vi "Overlay GD & T.vi"(8 "error in (no error)":errorcluster, 10 "Overlay details in":T1, 11 "Image in":T2) -> (0 "error out":errorcluster, 1 "Overlay coordinates":cluster{"X":dbl, "Y":dbl}[](array[cluster]), 2 "Text origin":cluster{"X":dbl, "Y":dbl}, 3 "Image out":T2)   [LabVIEW 2019]
uses:
  <vilib>/vision/Image Controls.llb/IMAQ Image.ctl
  Controls/GD&T overlay.ctl
  <vilib>/vision/NI_Vision_Development_Module.lvlib
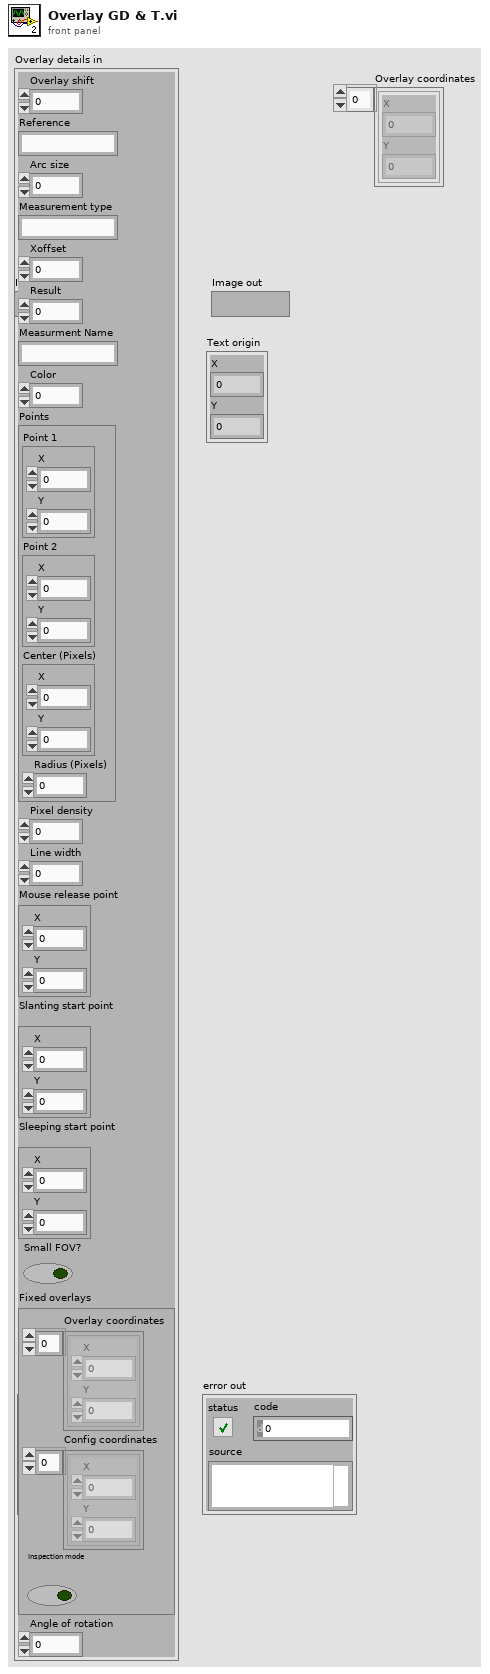
[diagram p1: front panel]
types:
  T1 = typedef "GD&T overlay.ctl" = cluster{"Overlay shift":dbl, "Reference":string, "Arc size":dbl, "Measurement type":string, "Xoffset":i32, "Result":sgl, "Measurment Name":string, "Color":u32, "Points":cluster{"Point 1":cluster{"X":sgl, "Y":sgl}, "Point 2":cluster{"X":sgl, "Y":sgl}, "Center (Pixels)":cluster{"X":sgl, "Y":sgl}, "Radius (Pixels)":dbl}, "Pixel density":dbl, "Line width":i32, "Mouse release point":cluster{"X":dbl, "Y":dbl}, "Slanting start point":cluster{"X":dbl, "Y":dbl}, "Sleeping start point":cluster{"X":dbl, "Y":dbl}, "Small FOV?":bool, "Fixed overlays":cluster{"Overlay coordinates":cluster{"X":dbl, "Y":dbl}[], "Config coordinates":cluster{"X":dbl, "Y":dbl}[], "Inspection mode":bool}, "Angle of rotation":dbl}
  T2 = typedef "IMAQ Image.ctl" = refnum<image>
  T3 = cluster{"Point 1":cluster{"X":sgl, "Y":sgl}, "Point 2":cluster{"X":sgl, "Y":sgl}}
  T4 = cluster{"Point 1":cluster{"X":sgl, "Y":sgl}, "Point 2":cluster{"X":sgl, "Y":sgl}, "Center (Pixels)":cluster{"X":sgl, "Y":sgl}, "Radius (Pixels)":dbl}
  T5 = cluster{"Feature":cluster{"X":dbl, "Y":dbl}[], "Directing points":cluster{"X":dbl, "Y":dbl}[], "Bounding box (symbols)":cluster{"X":dbl, "Y":dbl}[], "Symbols":cluster{"X":dbl, "Y":dbl}[], "Bounding box (Results)":cluster{"X":dbl, "Y":dbl}[], "Results":cluster{"X":dbl, "Y":dbl}[], "Bounding box (Reference)":cluster{"X":dbl, "Y":dbl}[], "Reference":cluster{"X":dbl, "Y":dbl}[]}
  T6 = cluster{"Center (Pixels)":cluster{"X":sgl, "Y":sgl}, "Radius (Pixels)":dbl}
  T7 = cluster{"Overlay coordinates":cluster{"X":dbl, "Y":dbl}[], "Config coordinates":cluster{"X":dbl, "Y":dbl}[], "Inspection mode":bool}
  T8 = cluster{"Overlay coordinates":cluster{"X":dbl, "Y":dbl}[], "Config coordinates":cluster{"X":dbl, "Y":dbl}[], "Inspection mode?":bool}
  T9 = enum16{"User-specified Font", "Application Font", "System Font", "Dialog Font"}
  T10 = cluster{"Desired Font (Application)":enum16{"User-specified Font", "Application Font", "System Font", "Dialog Font"}, "[User-specified Font]":cluster{"Font Name":string, "Size":i16, "Strikeout?":bool, "Italic?":bool, "Underline?":bool, "Outline?":bool, "Shadow?":bool, "Bold?":bool, "Rotation Angle":dbl}, "Horizontal Alignment":i16, "Vertical Alignment":i16}
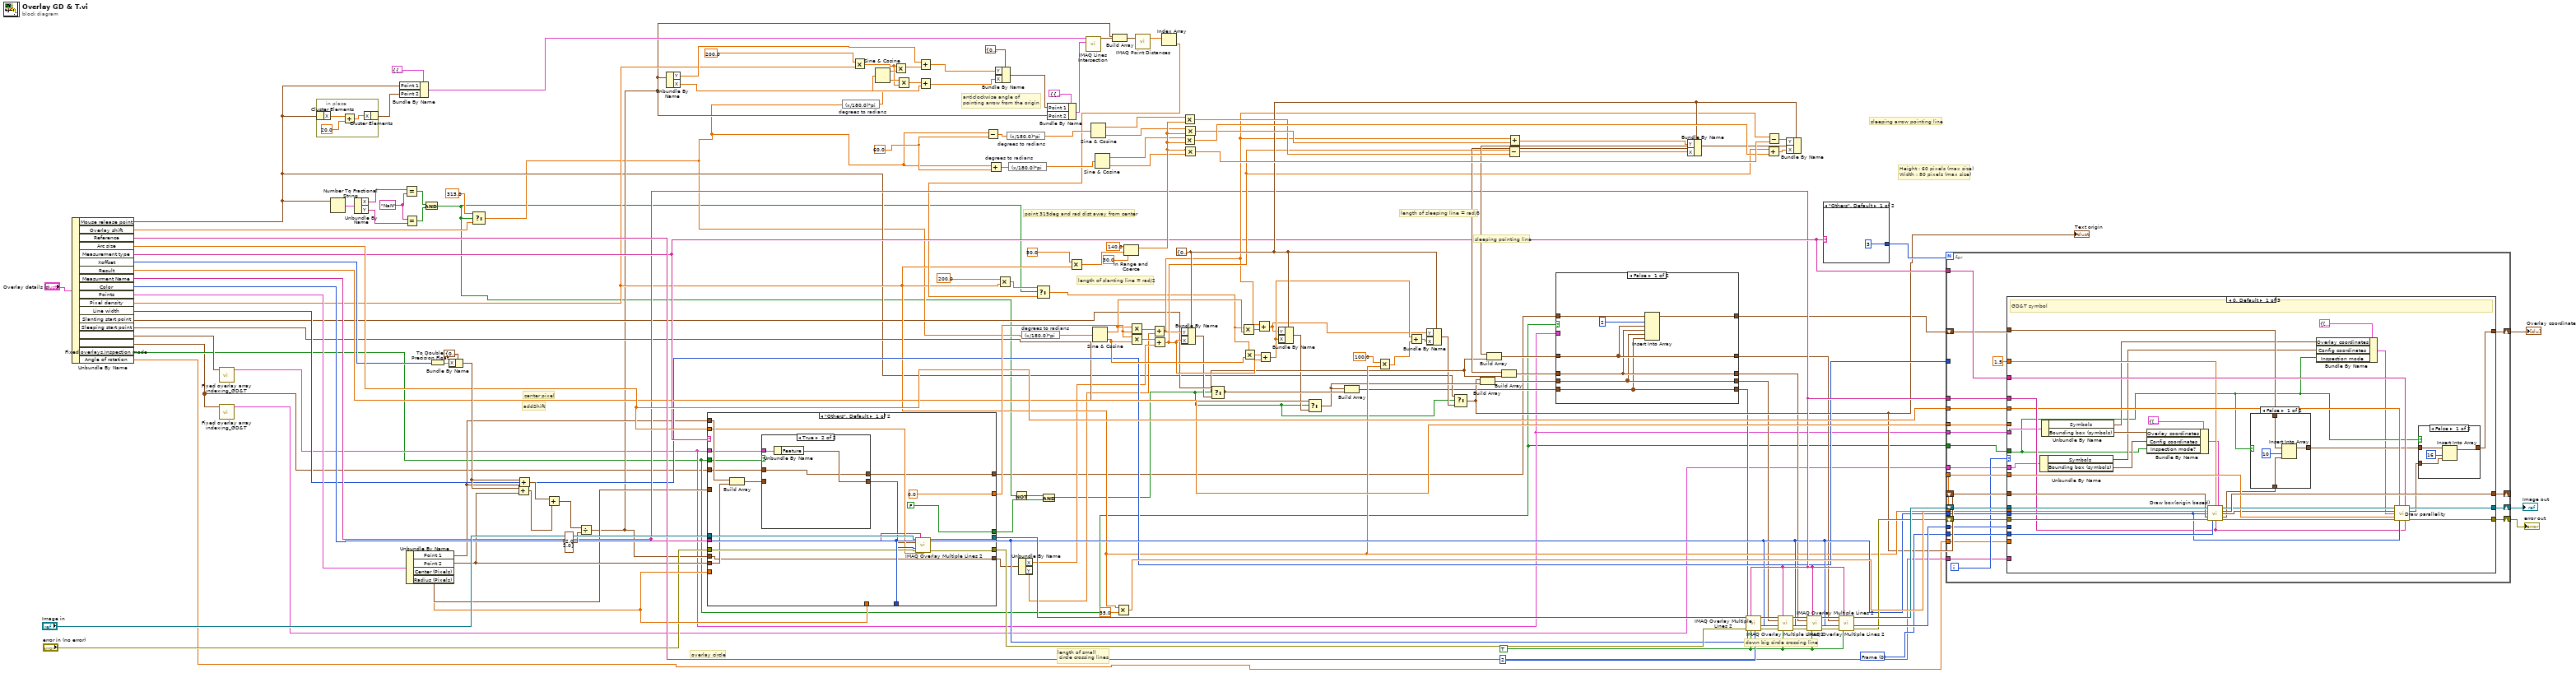
[diagram p0: block diagram]
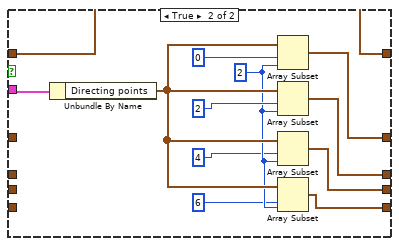
[diagram p2: hidden frame]
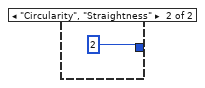
[diagram p3: hidden frame]
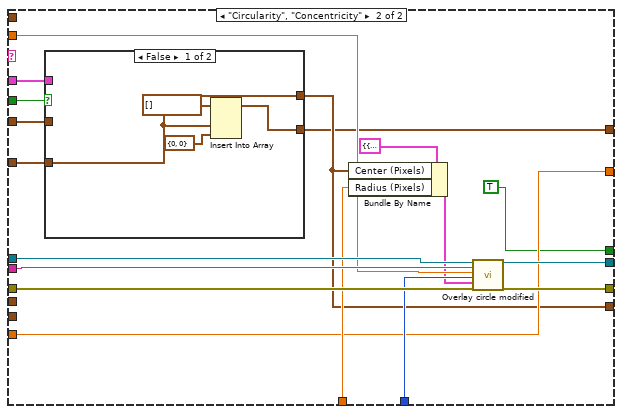
[diagram p5: hidden frame]
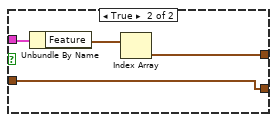
[diagram p6: hidden frame]
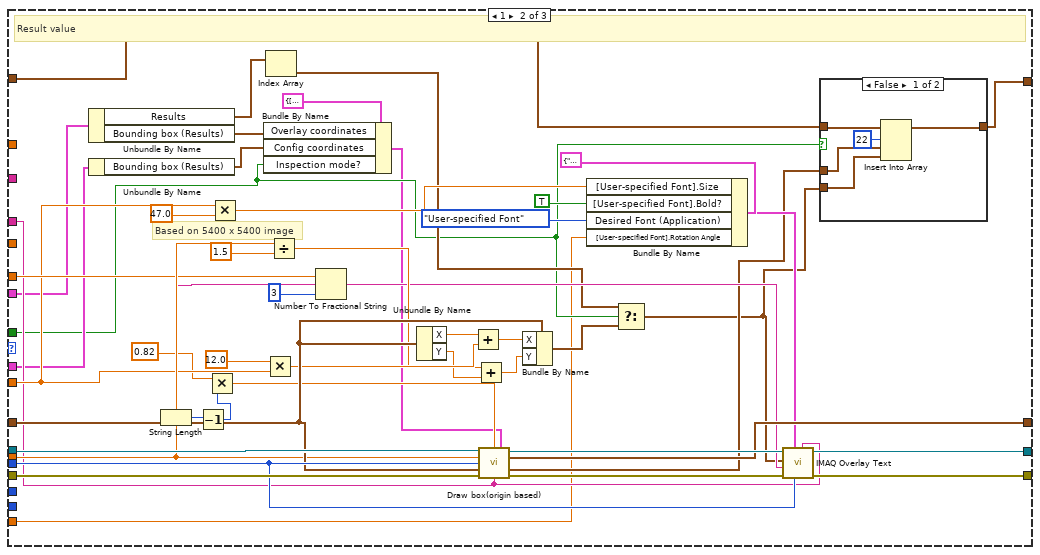
[diagram p9: hidden frame]
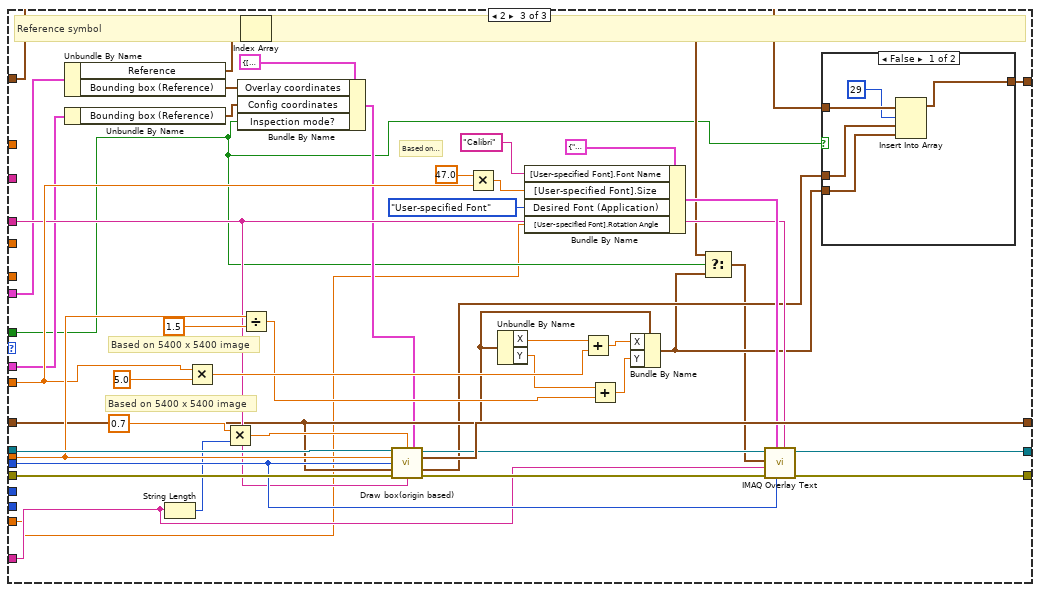
[diagram p11: hidden frame]
diagram:
  w71 = "NaN" ("y")
  w150 = u32 2 ("Width")
  w149 = TRUE ("Maintain Width?")
  w117 = 60.0
  w106 = u32 0 items=["Frame", "Fill"] ("Drawing Mode (Frame)")
  w132 = cluster{"X":sgl, "Y":sgl} {"X"=0.0, "Y"=0.0} ("Point 1")
  # "Height : 60 pixels (max size)\nWidth : 80 pixels (max size)"
  # "length of sleeping line = rad/8"
  # "point 315deg and rad dist away from center"
  # "length of slanting line = rad/2"
  # "length of small\n circle crossing lines"
  # "anticlockwise angle of\npointing arrow from the origin"
  # "sleeping arrow pointing line"
  # "sleeping pointing line"
  # "down big circle crossing line"
  # "addShift"
  # "center pixel"
  # "overlay circle"
  n1 = Unbundle By Name("Overlay details in") -> ("Mouse release point"=w26:cluster{"X":dbl, "Y":dbl}, "Overlay shift"=w21:dbl, "Reference"=w83:string, "Arc size"=w82:dbl, "Measurement type"=w81:string, "Xoffset"=w80:i32, "Result"=w79:sgl, "Measurment Name"=w78:string, "Color"=w77:u32, "Points"=w76:T4, "Pixel density"=w43:dbl, "Line width"=w75:i32, "Slanting start point"=w41:cluster{"X":dbl, "Y":dbl}, "Sleeping start point"=w38:cluster{"X":dbl, "Y":dbl}, "Fixed overlays.Overlay coordinates"=w17:cluster{"X":dbl, "Y":dbl}[], "Fixed overlays.Config coordinates"=w5:cluster{"X":dbl, "Y":dbl}[], "Fixed overlays.Inspection mode"=w6:bool, "Angle of rotation"=w1:dbl)
  n2 = call "Fixed overlay array indexing_GD&T.vi"("Overlay coordinates"=w17) -> ("Overlay coordinates cluster"=w7:T5)  [unwired: 10 in]
  n3 = call "Fixed overlay array indexing_GD&T.vi"("Overlay coordinates"=w5) -> ("Overlay coordinates cluster"=w4:T5)  [unwired: 10 in]
  n4 = in-place {
    n5 = in-place-cluster #1(w26) -> ("X"=w153:dbl)
    n6 = Add(x=w153, y=20.0) -> (x+y=w151:dbl)
    n7 = in-place-cluster #1("X"=w151) -> (w66:cluster{"X":dbl, "Y":dbl})
  }
  n8 = Number To Fractional String(number=w26) -> (F-format string=w74:cluster{"X":string, "Y":string})  [unwired: 3 in]
  n9 = Unbundle By Name(w74) -> ("X"=w73:string, "Y"=w72:string)
  n10 = Bundle By Name(cluster=T3 {"Point 1"={"X"=0.0, "Y"=0.0}, "Point 2"={"X"=0.0, "Y"=0.0}} ("Line 1"), "Point 1"=w26, "Point 2"=w66) -> (w65:T3)
  n11 = Equal?(x=w73, y=w71) -> (x = y?=w70:bool)
  n12 = Equal?(x=w71, y=w72) -> (x = y?=w69:bool)
  n13 = Unbundle By Name(w76) -> ("Point 1"=w68:cluster{"X":sgl, "Y":sgl}, "Point 2"=w35:cluster{"X":sgl, "Y":sgl}, "Center (Pixels)"=w34:cluster{"X":sgl, "Y":sgl}, "Radius (Pixels)"=w33:dbl)
  n14 = And(x=w70, y=w69) -> (x .and. y?=w19:bool)
  n15 = To Double Precision Float(number=w80) -> (double precision float=w97:dbl)
  n16 = Bundle By Name(cluster=cluster{"X":sgl, "Y":sgl} {"X"=0.0, "Y"=0.0} ("Angle.Point 2a"), "X"=w97) -> (w98:cluster{"X":sgl, "Y":sgl})
  n17 = Select(t=315.0, s=w19, f=w21) -> (s? t:f=w20:dbl)
  n18 = Add(x=w98, y=w35) -> (x+y=w102:cluster{"X":sgl, "Y":sgl})
  n19 = Add(x=w98, y=w68) -> (x+y=w101:cluster{"X":sgl, "Y":sgl})
  n20 = Add(x=w101, y=w102) -> (x+y=w99:cluster{"X":sgl, "Y":sgl})
  n21 = Divide(x=w99, y=cluster{"X":sgl, "Y":sgl} {"X"=2.0, "Y"=2.0}) -> (x/y=w28:cluster{"X":sgl, "Y":sgl})
  n22 = Unbundle By Name(w28) -> ("Y"=w61:sgl, "X"=w56:sgl)
  n23 = case shown="\"Others\", Default" w81 {
    tunnel: w33 -> [_ w183]
    tunnel: [sgl 0.0 w183] -> w116
    tunnel: "error in (no error)" -> [w171 w193]
    tunnel: [w170 w192] -> w146
    tunnel: "Image in" -> [w168 w191]
    tunnel: [w167 w190] -> w148
    tunnel: w78 -> [w163 w189]
    tunnel: w82 -> [w164 w188]
    tunnel: w77 -> [w169 w187]
    tunnel: w34 -> [_ w181]
    tunnel: w33 -> [_ w185]
    tunnel: w68 -> [w166 _]
    tunnel: w35 -> [w165 _]
    tunnel: [FALSE TRUE] -> w24
    tunnel: w28 -> [w160 _]
    tunnel: [w160 w180] -> w31
    tunnel: w6 -> [w157 w179]
    tunnel: w7 -> [w155 w178]
    tunnel: w5 -> [w154 w177]
    tunnel: [w156 w176] -> w8
    frame "Others", Default {
      n24 = Build Array(w166, w165) -> (w159:cluster{"X":sgl, "Y":sgl}[])
      n25 = case shown="True" w157 {
        tunnel: w159 -> [w172 _]
        tunnel: [w172 w174] -> w158
        tunnel: [w172 w173] -> w156
        tunnel: w155 -> [_ w175]
        tunnel: w154 -> [_ w173]
        frame False {
        }
        frame True {
          n26 = Unbundle By Name(w175) -> ("Feature"=w174:cluster{"X":dbl, "Y":dbl}[])
        }
      }
      n27 = call "IMAQ Overlay Multiple Lines 2"("Image"=w168, "Group"=w163, "Line End Points"=w158, "Color"=w169, "error in (no error)"=w171, "Width"=w164) -> ("Image Out"=w167:T2, "error out"=w170:errorcluster)  [unwired: 8 in]
    }
    frame "Circularity", "Concentricity" {
      n28 = case shown="False" w179 {
        tunnel: w181 -> [w197 _]
        tunnel: [w197 w199] -> w180
        tunnel: w178 -> [_ w201]
        tunnel: [w195 w198] -> w176
        tunnel: w177 -> [_ w198]
        frame False {
          n29 = Insert Into Array(array=cluster{"X":sgl, "Y":sgl}[] [], new element #1=w197, new element #2=cluster{"X":i32, "Y":i32} {"X"=0, "Y"=0} ("Center (Pixels)")) -> (w195:cluster{"X":sgl, "Y":sgl}[])  [unwired: 1 in]
        }
        frame True {
          n30 = Unbundle By Name(w201) -> ("Feature"=w200:cluster{"X":dbl, "Y":dbl}[])
          n31 = Index Array(array=w200) -> (element=w199:cluster{"X":dbl, "Y":dbl})  [unwired: 1 in]
        }
      }
      n32 = Bundle By Name(cluster=T6 {"Center (Pixels)"={"X"=0.0, "Y"=0.0}, "Radius (Pixels)"=0.0} ("Circle center"), "Center (Pixels)"=w180, "Radius (Pixels)"=w185) -> (w184:T6)
      n33 = call "Overlay circle modified.vi"("Image In"=w191, "Measurment Name"=w189, "Overlay width"=w188, "Overlay color"=w187, "Circle center"=w184, "error in (no error)"=w193) -> ("Image out"=w190:T2, "error out"=w192:errorcluster)  [unwired: 12 in]
    }
  }
  n34 = expression code="(x/180.0)*pi" "degrees to radians"(w20) -> (w47:dbl)
  n35 = Multiply(x=sgl 200.0, y=w43) -> (x*y=w58:dbl)
  n36 = Sine & Cosine(0:w47) -> (1:w62:dbl, 2:w59:dbl)
  n37 = Multiply(x=w58, y=w62) -> (x*y=w60:dbl)
  n38 = Multiply(x=w59, y=w58) -> (x*y=w57:dbl)
  n39 = Add(x=w61, y=w60) -> (x+y=w54:dbl)
  n40 = Add(x=w57, y=w56) -> (x+y=w53:dbl)
  n41 = Subtract(x=w20, y=w117) -> (x-y=w118:dbl)
  n42 = Add(x=w20, y=w117) -> (x+y=w119:dbl)
  n43 = Bundle By Name(cluster=cluster{"X":sgl, "Y":sgl} {"X"=0.0, "Y"=0.0} ("x/y"), "Y"=w54, "X"=w53) -> (w52:cluster{"X":sgl, "Y":sgl})
  n44 = Multiply(x=200.0 ("t"), y=w43) -> (x*y=w42:dbl)
  n45 = expression code="(x/180.0)*pi" "degrees to radians"(w118) -> (w124:dbl)
  n46 = expression code="(x/180.0)*pi" "degrees to radians"(w119) -> (w125:dbl)
  n47 = Not(x=w19) -> (.not. x?=w18:bool)
  n48 = Unbundle By Name(w31) -> ("X"=w30:dbl, "Y"=w29:dbl)
  n49 = expression code="(x/180.0)*pi" "degrees to radians"(w20) -> (w85:dbl)
  n50 = And(x=w18, y=w24) -> (x .and. y?=w23:bool)
  n51 = Bundle By Name(cluster=T3 {"Point 1"={"X"=0.0, "Y"=0.0}, "Point 2"={"X"=0.0, "Y"=0.0}} ("Line 1"), "Point 1"=w52, "Point 2"=w28) -> (w51:T3)
  n52 = Multiply(x=sgl 50.0, y=w43) -> (x*y=w141:dbl)
  n53 = call "IMAQ Lines Intersection"("Line 2"=w51, "Line 1"=w65) -> ("Intersection Point"=w50:cluster{"X":sgl, "Y":sgl})  [unwired: 7 in, 2 out]
  n54 = Sine & Cosine(0:w124) -> (1:w120:dbl, 2:w121:dbl)
  n55 = Sine & Cosine(0:w85) -> (1:w86:dbl, 2:w87:dbl)
  n56 = Sine & Cosine(0:w125) -> (1:w122:dbl, 2:w123:dbl)
  n57 = Build Array(w28, w50) -> (w49:cluster{"X":sgl, "Y":sgl}[])
  n58 = Multiply(x=w43, y=35.0) -> (x*y=w107:dbl)
  n59 = In Range and Coerce(upper limit=140.0, x=w141, lower limit=30.0) -> (coerced(x)=w144:dbl)  [unwired: 1 out]
  n60 = Multiply(x=w86, y=w116) -> (x*y=w94:dbl)
  n61 = Multiply(x=w116, y=w87) -> (x*y=w95:dbl)
  n62 = call "IMAQ Point Distances"("Points"=w49) -> ("Distances"=w48:sgl[])  [unwired: 4 in, 1 out]
  n63 = Add(x=w94, y=w29) -> (x+y=w130:dbl)
  n64 = Add(x=w95, y=w30) -> (x+y=w131:dbl)
  n65 = Index Array(array=w48) -> (element=w45:sgl)  [unwired: 1 in]
  n66 = Select(t=w42, s=w19, f=w45) -> (s? t:f=w46:dbl)
  n67 = Bundle By Name(cluster=w132, "Y"=w130, "X"=w131) -> (w40:cluster{"X":sgl, "Y":sgl})
  n68 = Multiply(x=w120, y=w144) -> (x*y=w135:dbl)
  n69 = Multiply(x=w122, y=w144) -> (x*y=w137:dbl)
  n70 = Multiply(x=w121, y=w144) -> (x*y=w136:dbl)
  n71 = Multiply(x=w144, y=w123) -> (x*y=w138:dbl)
  n72 = Select(t=w41, s=w23, f=w40) -> (s? t:f=w39:cluster{"X":dbl, "Y":dbl})
  n73 = Multiply(x=w46, y=w86) -> (x*y=w88:dbl)
  n74 = Multiply(x=w46, y=w87) -> (x*y=w89:dbl)
  n75 = Add(x=w130, y=w88) -> (x+y=w92:dbl)
  n76 = Add(x=w89, y=w131) -> (x+y=w93:dbl)
  n77 = Bundle By Name(cluster=w132, "Y"=w92, "X"=w93) -> (w37:cluster{"X":sgl, "Y":sgl})
  n78 = Select(t=w38, s=w23, f=w37) -> (s? t:f=w36:cluster{"X":dbl, "Y":dbl})
  n79 = Build Array(w36, w39) -> (w10:cluster{"X":dbl, "Y":dbl}[])
  n80 = Multiply(x=100.0, y=w43) -> (x*y=w90:dbl)
  n81 = Add(x=w93, y=w90) -> (x+y=w91:dbl)
  n82 = Bundle By Name(cluster=w132, "Y"=w92, "X"=w91) -> (w27:cluster{"X":sgl, "Y":sgl})
  n83 = Select(t=w26, s=w23, f=w27) -> (s? t:f=w25:cluster{"X":dbl, "Y":dbl})
  "Text origin" <- w25
  n84 = Build Array(w25, w36) -> (w12:cluster{"X":dbl, "Y":dbl}[])
  n85 = Subtract(x=w131, y=w135) -> (x-y=w126:dbl)
  n86 = Add(x=w130, y=w136) -> (x+y=w128:dbl)
  n87 = Bundle By Name(cluster=w132, "Y"=w128, "X"=w126) -> (w133:cluster{"X":sgl, "Y":sgl})
  n88 = Build Array(w133, w39) -> (w14:cluster{"X":dbl, "Y":dbl}[])
  n89 = Add(x=w131, y=w137) -> (x+y=w129:dbl)
  n90 = Subtract(x=w130, y=w138) -> (x-y=w127:dbl)
  n91 = Bundle By Name(cluster=w132, "Y"=w127, "X"=w129) -> (w134:cluster{"X":sgl, "Y":sgl})
  n92 = Build Array(w134, w39) -> (w16:cluster{"X":dbl, "Y":dbl}[])
  n93 = case shown="False" w6 {
    tunnel: w16 -> [w207 _]
    tunnel: [w207 w213] -> w15
    tunnel: w14 -> [w206 _]
    tunnel: [w206 w212] -> w13
    tunnel: w12 -> [w205 _]
    tunnel: [w205 w211] -> w11
    tunnel: w10 -> [w204 _]
    tunnel: [w204 w210] -> w9
    tunnel: w7 -> [_ w220]
    tunnel: w8 -> [w208 w209]
    tunnel: [w203 w209] -> w3
    frame False {
      n94 = Insert Into Array(array=w208, index=2, new element #1=w207, new element #2=w206, new element #3=w205, new element #4=w204) -> (w203:cluster{"X":dbl, "Y":dbl}[])
    }
    frame True {
      w216 = 2 ("length")
      n95 = Unbundle By Name(w220) -> ("Directing points"=w219:cluster{"X":dbl, "Y":dbl}[])
      n96 = Array Subset(array=w219, index=0, length=w216) -> (w213:cluster{"X":dbl, "Y":dbl}[])
      n97 = Array Subset(array=w219, index=2, length=w216) -> (w212:cluster{"X":dbl, "Y":dbl}[])
      n98 = Array Subset(array=w219, index=4, length=w216) -> (w211:cluster{"X":dbl, "Y":dbl}[])
      n99 = Array Subset(array=w219, index=6, length=w216) -> (w210:cluster{"X":dbl, "Y":dbl}[])
    }
  }
  n100 = call "IMAQ Overlay Multiple Lines 2"("Image"=w148, "Group"=w78, "Line End Points"=w9, "Color"=w77, "error in (no error)"=w146, "Maintain Width?"=w149, "Width"=w150) -> ("Image Out"=w111:T2, "error out"=w110:errorcluster)  [unwired: 7 in]
  n101 = call "IMAQ Overlay Multiple Lines 2"("Image"=w111, "Group"=w78, "Line End Points"=w11, "Color"=w77, "error in (no error)"=w110, "Maintain Width?"=w149, "Width"=w150) -> ("Image Out"=w113:T2, "error out"=w112:errorcluster)  [unwired: 7 in]
  n102 = call "IMAQ Overlay Multiple Lines 2"("Image"=w113, "Group"=w78, "Line End Points"=w13, "Color"=w77, "error in (no error)"=w112, "Maintain Width?"=w149, "Width"=w150) -> ("Image Out"=w114:T2, "error out"=w115:errorcluster)  [unwired: 7 in]
  n103 = case shown="\"Others\", Default" w81 {
    tunnel: [3 2] -> w145
    frame "Others", Default {
    }
    frame "Circularity", "Straightness" {
    }
  }
  n104 = call "IMAQ Overlay Multiple Lines 2"("Image"=w114, "Group"=w78, "Line End Points"=w15, "Color"=w77, "error in (no error)"=w115, "Maintain Width?"=w149, "Width"=w150) -> ("Image Out"=w105:T2, "error out"=w103:errorcluster)  [unwired: 7 in]
  n105 = for {
    N: w145 -> [_]
    tunnel: w150 -> [w236]
    tunnel: w106 -> [w244]
    tunnel: w107 -> [w240]
    tunnel: w77 -> [w238]
    shift-right: [w241] -> w104
    shift-left: w103 -> [w246]
    shift-right: [w239] -> w108
    shift-left: w105 -> [w245]
    shift-right: [w243] -> _
    shift-left: w25 -> [w242]
    tunnel: w43 -> [w237]
    tunnel: w79 -> [w234]
    tunnel: w81 -> [w233]
    tunnel: w83 -> [w232]
    tunnel: w78 -> [w231]
    tunnel: w82 -> [w230]
    tunnel: w75 -> [_]
    tunnel: w7 -> [w228]
    tunnel: w6 -> [w227]
    tunnel: w4 -> [w226]
    shift-right: [w225] -> w2
    shift-left: w3 -> [w224]
    tunnel: w1 -> [w223]
    i -> [w235]
    n106 = case shown="0, Default" w235 {
      tunnel: w246 -> [w279 w337 w388]
      tunnel: w245 -> [w278 w336 w387]
      tunnel: w244 -> [w277 _ _]
      tunnel: [w276 w324 w386] -> w243
      tunnel: w242 -> [w275 w330 w359]
      tunnel: [w273 w334 w384] -> w241
      tunnel: w240 -> [w272 w321 w376]
      tunnel: [w270 w332 w382] -> w239
      tunnel: w238 -> [w269 w331 w381]
      tunnel: w237 -> [w268 w314 w364]
      tunnel: w236 -> [_ _ _]
      tunnel: w234 -> [_ w316 _]
      tunnel: w233 -> [w267 _ _]
      tunnel: w232 -> [_ _ w363]
      tunnel: w231 -> [w266 w312 w362]
      tunnel: w230 -> [w265 _ _]
      tunnel: 1.5 ("Line width") -> [w264 _ _]
      tunnel: w228 -> [w262 w304 w358]
      tunnel: w227 -> [w248 w298 w345]
      tunnel: w224 -> [w259 w294 w347]
      tunnel: w226 -> [w255 w301 w355]
      tunnel: [w253 w293 w346] -> w225
      tunnel: w223 -> [_ w290 w344]
      frame 0, Default {
        # "GD&T symbol"
        n107 = Unbundle By Name(w255) -> ("Symbols"=w249:cluster{"X":dbl, "Y":dbl}[], "Bounding box (symbols)"=w254:cluster{"X":dbl, "Y":dbl}[])
        n108 = Unbundle By Name(w262) -> ("Symbols"=w250:cluster{"X":dbl, "Y":dbl}[], "Bounding box (symbols)"=w261:cluster{"X":dbl, "Y":dbl}[])
        n109 = Bundle By Name(cluster=T8 {"Overlay coordinates"=[{"X"=1328.0, "Y"=1221.0}, {"X"=1324.0, "Y"=1190.0}, {"X"=1386.0, "Y"=1180.0}, {"X"=1391.0, "Y"=1211.0}, {"X"=1328.0, "Y"=1221.0}, {"X"=1355.0, "Y"=1185.0}, {"X"=1381.0, "Y"=1212.0}, {"X"=1156.0, "Y"=1497.0}, {"X"=1115.0, "Y"=1492.0}, {"X"=1163.0, "Y"=1538.0}, {"X"=1156.0, "Y"=1497.0}, {"X"=1370.0, "Y"=1278.0}, {"X"=1360.0, "Y"=1216.0}, {"X"=1382.0, "Y"=1751.0}, {"X"=896.0, "Y"=1279.0}], "Config coordinates"=[{"X"=1892.1014404296875, "Y"=1412.35791015625}, {"X"=1923.478515625, "Y"=1412.35791015625}, {"X"=1923.478515625, "Y"=1475.112060546875}, {"X"=1892.1014404296875, "Y"=1475.112060546875}, {"X"=1892.1014404296875, "Y"=1412.35791015625}, {"X"=1923.478515625, "Y"=1443.7349853515625}, {"X"=1892.143310546875, "Y"=1464.653076171875}, {"X"=1646.9659423828125, "Y"=1198.1522216796875}, {"X"=1658.86962890625, "Y"=1158.0452880859375}, {"X"=1605.13037109375, "Y"=1197.9547119140625}, {"X"=1646.9659423828125, "Y"=1198.1522216796875}, {"X"=1829.3472900390625, "Y"=1443.7349853515625}, {"X"=1892.1014404296875, "Y"=1443.7349853515625}, {"X"=1360.0, "Y"=1380.0}, {"X"=1904.0, "Y"=976.0}], "Inspection mode?"=TRUE} ("Fixed overlay details"), "Overlay coordinates"=w261, "Config coordinates"=w254, "Inspection mode?"=w248) -> (w263:T8)
        n110 = call "Draw box(origin based).vi"("Image"=w278, "Width factor"=w264, "Fixed overlay details"=w263, "Size bias factor"=w272, "Color Box"=w269, "Origin"=w275, "error in (no error)"=w279, "Drawing Mode (Frame)"=w277, "Group name"=w266) -> ("Image Out"=w271:T2, "Right adjacent origin"=w276:cluster{"X":sgl, "Y":sgl}, "Bounding rectangle array"=w260:cluster{"X":dbl, "Y":dbl}[], "Overlay coordinates out"=w256:cluster{"X":dbl, "Y":dbl}[], "error out"=w274:errorcluster)  [unwired: 2 in]
        n111 = case shown="False" w248 {
          tunnel: w256 -> [w288 _]
          tunnel: w259 -> [w287 w289]
          tunnel: [w286 w289] -> w258
          frame False {
            n112 = Insert Into Array(array=w287, index=10, new element=w288) -> (w286:cluster{"X":dbl, "Y":dbl}[])
          }
          frame True {
          }
        }
        n113 = Bundle By Name(cluster=T7 {"Overlay coordinates"=[], "Config coordinates"=[], "Inspection mode"=FALSE} ("Fixed overlay in"), "Overlay coordinates"=w250, "Config coordinates"=w249, "Inspection mode"=w248) -> (w247:T7)
        n114 = call "Draw parallelity.vi"("Image in"=w271, "Arc width"=w265, "Overlay type"=w267, "Bounding rectangle array"=w260, "Fixed overlay in"=w247, "Size factor"=w268, "error in (no error)"=w274, "Overlay color"=w269, "Measurment Name"=w266) -> ("Image Out"=w270:T2, "Overlay coordinates"=w257:cluster{"X":dbl, "Y":dbl}[], "error out"=w273:errorcluster)  [unwired: 4 in]
        n115 = case shown="False" w248 {
          tunnel: w258 -> [w283 w284]
          tunnel: [w280 w284] -> w253
          tunnel: w257 -> [w281 _]
          frame False {
            n116 = Insert Into Array(array=w283, index=16, new element=w281) -> (w280:cluster{"X":dbl, "Y":dbl}[])
          }
          frame True {
          }
        }
      }
      frame 1 {
        # "Based on 5400 x 5400 image"
        # "Result value"
        n117 = Unbundle By Name(w304) -> ("Results"=w300:cluster{"X":dbl, "Y":dbl}[], "Bounding box (Results)"=w303:cluster{"X":dbl, "Y":dbl}[])
        n118 = Unbundle By Name(w301) -> ("Bounding box (Results)"=w302:cluster{"X":dbl, "Y":dbl}[])
        n119 = Multiply(x=w314, y=sgl 47.0) -> (x*y=w305:dbl)
        n120 = Bundle By Name(cluster=T8 {"Overlay coordinates"=[{"X"=1328.0, "Y"=1221.0}, {"X"=1324.0, "Y"=1190.0}, {"X"=1386.0, "Y"=1180.0}, {"X"=1391.0, "Y"=1211.0}, {"X"=1328.0, "Y"=1221.0}, {"X"=1355.0, "Y"=1185.0}, {"X"=1381.0, "Y"=1212.0}, {"X"=1156.0, "Y"=1497.0}, {"X"=1115.0, "Y"=1492.0}, {"X"=1163.0, "Y"=1538.0}, {"X"=1156.0, "Y"=1497.0}, {"X"=1370.0, "Y"=1278.0}, {"X"=1360.0, "Y"=1216.0}, {"X"=1382.0, "Y"=1751.0}, {"X"=896.0, "Y"=1279.0}], "Config coordinates"=[{"X"=1892.1014404296875, "Y"=1412.35791015625}, {"X"=1923.478515625, "Y"=1412.35791015625}, {"X"=1923.478515625, "Y"=1475.112060546875}, {"X"=1892.1014404296875, "Y"=1475.112060546875}, {"X"=1892.1014404296875, "Y"=1412.35791015625}, {"X"=1923.478515625, "Y"=1443.7349853515625}, {"X"=1892.143310546875, "Y"=1464.653076171875}, {"X"=1646.9659423828125, "Y"=1198.1522216796875}, {"X"=1658.86962890625, "Y"=1158.0452880859375}, {"X"=1605.13037109375, "Y"=1197.9547119140625}, {"X"=1646.9659423828125, "Y"=1198.1522216796875}, {"X"=1829.3472900390625, "Y"=1443.7349853515625}, {"X"=1892.1014404296875, "Y"=1443.7349853515625}, {"X"=1360.0, "Y"=1380.0}, {"X"=1904.0, "Y"=976.0}], "Inspection mode?"=TRUE} ("Fixed overlay details"), "Overlay coordinates"=w303, "Config coordinates"=w302, "Inspection mode?"=w298) -> (w291:T8)
        n121 = Multiply(x=12.0, y=w314) -> (x*y=w326:dbl)
        n122 = Index Array(array=w300) -> (element=w299:cluster{"X":dbl, "Y":dbl})  [unwired: 1 in]
        n123 = Divide(x=w321, y=1.5) -> (x/y=w319:dbl)
        n124 = Number To Fractional String(number=w316, precision (6)=i16 3) -> (F-format string=w310:string)  [unwired: 2 in]
        n125 = String Length(string=w310) -> (length=w309:i32)
        n126 = Decrement(x=w309) -> (x-1=w308:i32)
        n127 = Multiply(x=0.82 ("Width factor"), y=w308) -> (x*y=w307:dbl)
        n128 = Unbundle By Name(w330) -> ("X"=w329:dbl, "Y"=w323:dbl)
        n129 = Add(x=w329, y=w326) -> (x+y=w328:dbl)
        n130 = Add(x=w319, y=w323) -> (x+y=w322:dbl)
        n131 = call "Draw box(origin based).vi"("Image"=w336, "Width factor"=w307, "Fixed overlay details"=w291, "Size bias factor"=w321, "Color Box"=w331, "Origin"=w330, "error in (no error)"=w337, "Group name"=w312) -> ("Image Out"=w333:T2, "Right adjacent origin"=w324:cluster{"X":sgl, "Y":sgl}, "Overlay coordinates out"=w296:cluster{"X":dbl, "Y":dbl}[], "error out"=w335:errorcluster)  [unwired: 3 in, 1 out]
        n132 = Bundle By Name(cluster=w330, "X"=w328, "Y"=w322) -> (w297:cluster{"X":dbl, "Y":dbl})
        n133 = Bundle By Name(cluster=T10 {"Desired Font (Application)"=enum."User-specified Font", "[User-specified Font]"={"Font Name"="Calibri", "Size"=50, "Strikeout?"=FALSE, "Italic?"=FALSE, "Underline?"=FALSE, "Outline?"=FALSE, "Shadow?"=FALSE, "Bold?"=TRUE, "Rotation Angle"=0.0}, "Horizontal Alignment"=0, "Vertical Alignment"=0} ("Font, Size & Style"), "[User-specified Font].Size"=w305, "[User-specified Font].Bold?"=TRUE, "Desired Font (Application)"=T9."User-specified Font", "[User-specified Font].Rotation Angle"=w290) -> (w317:T10)
        n134 = Select(t=w299, s=w298, f=w297) -> (s? t:f=w295:cluster{"X":dbl, "Y":dbl})
        n135 = call "IMAQ Overlay Text"("Group"=w312, "Text Color (black)"=w331, "Font, Size & Style"=w317, "error in (no error)"=w335, "String"=w310, "Origin"=w295, "Image"=w333) -> ("error out"=w334:errorcluster, "Image Out"=w332:T2)  [unwired: 3 in]
        n136 = case shown="False" w298 {
          tunnel: w296 -> [w341 _]
          tunnel: w295 -> [w340 _]
          tunnel: w294 -> [w342 w343]
          tunnel: [w339 w343] -> w293
          frame False {
            n137 = Insert Into Array(array=w342, index=22, new element #1=w341, new element #2=w340) -> (w339:cluster{"X":dbl, "Y":dbl}[])
          }
          frame True {
          }
        }
      }
      frame 2 {
        # "Based on 5400 x 5400 image"
        # "Based on 5400 x 5400 image"
        # "Based on 5400 x 5400 image"
        # "Reference symbol"
        n138 = Unbundle By Name(w358) -> ("Reference"=w350:cluster{"X":dbl, "Y":dbl}[], "Bounding box (Reference)"=w354:cluster{"X":dbl, "Y":dbl}[])
        n139 = Unbundle By Name(w355) -> ("Bounding box (Reference)"=w356:cluster{"X":dbl, "Y":dbl}[])
        n140 = String Length(string=w363) -> (length=w371:i32)
        n141 = Multiply(x=w364, y=5.0) -> (x*y=w378:dbl)
        n142 = Multiply(x=0.7 ("Width factor"), y=w371) -> (x*y=w369:dbl)
        n143 = Bundle By Name(cluster=T8 {"Overlay coordinates"=[{"X"=1328.0, "Y"=1221.0}, {"X"=1324.0, "Y"=1190.0}, {"X"=1386.0, "Y"=1180.0}, {"X"=1391.0, "Y"=1211.0}, {"X"=1328.0, "Y"=1221.0}, {"X"=1355.0, "Y"=1185.0}, {"X"=1381.0, "Y"=1212.0}, {"X"=1156.0, "Y"=1497.0}, {"X"=1115.0, "Y"=1492.0}, {"X"=1163.0, "Y"=1538.0}, {"X"=1156.0, "Y"=1497.0}, {"X"=1370.0, "Y"=1278.0}, {"X"=1360.0, "Y"=1216.0}, {"X"=1382.0, "Y"=1751.0}, {"X"=896.0, "Y"=1279.0}], "Config coordinates"=[{"X"=1892.1014404296875, "Y"=1412.35791015625}, {"X"=1923.478515625, "Y"=1412.35791015625}, {"X"=1923.478515625, "Y"=1475.112060546875}, {"X"=1892.1014404296875, "Y"=1475.112060546875}, {"X"=1892.1014404296875, "Y"=1412.35791015625}, {"X"=1923.478515625, "Y"=1443.7349853515625}, {"X"=1892.143310546875, "Y"=1464.653076171875}, {"X"=1646.9659423828125, "Y"=1198.1522216796875}, {"X"=1658.86962890625, "Y"=1158.0452880859375}, {"X"=1605.13037109375, "Y"=1197.9547119140625}, {"X"=1646.9659423828125, "Y"=1198.1522216796875}, {"X"=1829.3472900390625, "Y"=1443.7349853515625}, {"X"=1892.1014404296875, "Y"=1443.7349853515625}, {"X"=1360.0, "Y"=1380.0}, {"X"=1904.0, "Y"=976.0}], "Inspection mode?"=TRUE} ("Fixed overlay details"), "Overlay coordinates"=w354, "Config coordinates"=w356, "Inspection mode?"=w345) -> (w353:T8)
        n144 = Index Array(array=w350) -> (element=w349:cluster{"X":dbl, "Y":dbl})  [unwired: 1 in]
        n145 = Divide(x=w376, y=1.5) -> (x/y=w373:dbl)
        n146 = call "Draw box(origin based).vi"("Image"=w387, "Width factor"=w369, "Fixed overlay details"=w353, "Size bias factor"=w376, "Color Box"=w381, "Origin"=w359, "error in (no error)"=w388, "Group name"=w362) -> ("Image Out"=w383:T2, "Right adjacent origin"=w386:cluster{"X":sgl, "Y":sgl}, "Overlay coordinates out"=w352:cluster{"X":dbl, "Y":dbl}[], "error out"=w385:errorcluster)  [unwired: 3 in, 1 out]
        n147 = Multiply(x=47.0, y=w364) -> (x*y=w367:dbl)
        n148 = Unbundle By Name(w359) -> ("X"=w380:dbl, "Y"=w374:dbl)
        n149 = Bundle By Name(cluster=T10 {"Desired Font (Application)"=enum."User-specified Font", "[User-specified Font]"={"Font Name"="Times New Roman", "Size"=45, "Strikeout?"=FALSE, "Italic?"=FALSE, "Underline?"=FALSE, "Outline?"=FALSE, "Shadow?"=FALSE, "Bold?"=TRUE, "Rotation Angle"=0.0}, "Horizontal Alignment"=0, "Vertical Alignment"=0} ("Font, Size & Style"), "[User-specified Font].Font Name"="Calibri", "[User-specified Font].Size"=w367, "Desired Font (Application)"=T9."User-specified Font", "[User-specified Font].Rotation Angle"=w344) -> (w365:T10)
        n150 = Add(x=w380, y=w378) -> (x+y=w377:dbl)
        n151 = Add(x=w374, y=w373) -> (x+y=w372:dbl)
        n152 = Bundle By Name(cluster=w359, "X"=w377, "Y"=w372) -> (w351:cluster{"X":dbl, "Y":dbl})
        n153 = Select(t=w349, s=w345, f=w351) -> (s? t:f=w348:cluster{"X":dbl, "Y":dbl})
        n154 = call "IMAQ Overlay Text"("Group"=w362, "Text Color (black)"=w381, "Font, Size & Style"=w365, "error in (no error)"=w385, "String"=w363, "Origin"=w348, "Image"=w383) -> ("error out"=w384:errorcluster, "Image Out"=w382:T2)  [unwired: 3 in]
        n155 = case shown="False" w345 {
          tunnel: w352 -> [w391 _]
          tunnel: w351 -> [w390 _]
          tunnel: w347 -> [w393 w394]
          tunnel: [w392 w394] -> w346
          frame False {
            n156 = Insert Into Array(array=w393, index=29, new element #1=w391, new element #2=w390) -> (w392:cluster{"X":dbl, "Y":dbl}[])
          }
          frame True {
          }
        }
      }
    }
  }
  "Image out" <- w108
  "error out" <- w104
  "Overlay coordinates" <- w2
